vi "TEST Object Manual Bounds (Advanced By Reference Splitter).vi"() -> ()   [LabVIEW 2021, in "IObject.lvclass"]
uses:
  IObject.lvclass
  Object/Object.lvclass
  C:/Projects/Dynamic-Scaling/Dynamic Scaling/IObject.lvclass
  IContainer/Viewport/Viewport.lvclass
  IContainer/Divider/Splitter/Splitter.lvclass
  Interaction By Refererence/Interaction By Refererence.lvclass
panel:
  out "XY Graph 6":cluster{"X":dbl, "Y":dbl}[](graph)
  out "XY Graph 5":cluster{"X":dbl, "Y":dbl}[](graph)
  out "XY Graph 4":cluster{"X":dbl, "Y":dbl}[](graph)
  out "XY Graph 3":cluster{"X":dbl, "Y":dbl}[](graph)
  out "XY Graph 2":cluster{"X":dbl, "Y":dbl}[](graph)
  out "XY Graph":cluster{"X":dbl, "Y":dbl}[](graph)
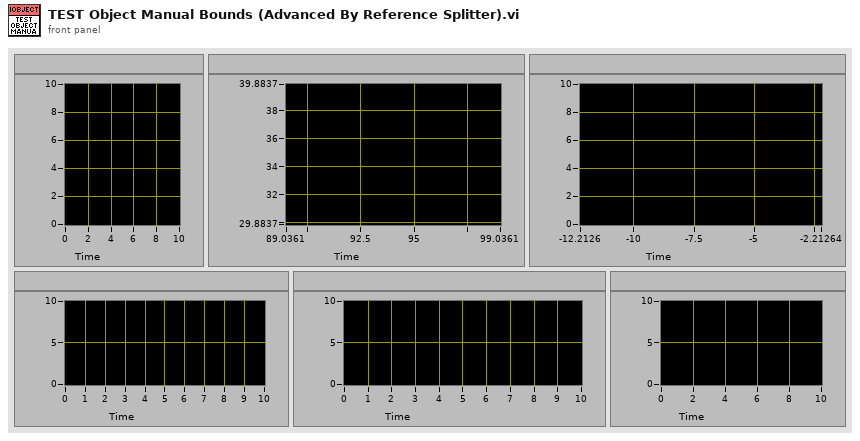
[diagram p1: front panel]
types:
  T1 = cluster{"Left":dbl, "Top":dbl, "Right":dbl, "Bottom":dbl}
  T2 = typedef "LVRectTypeDef.ctl" = cluster{"Left":i16, "Top":i16, "Right":i16, "Bottom":i16}
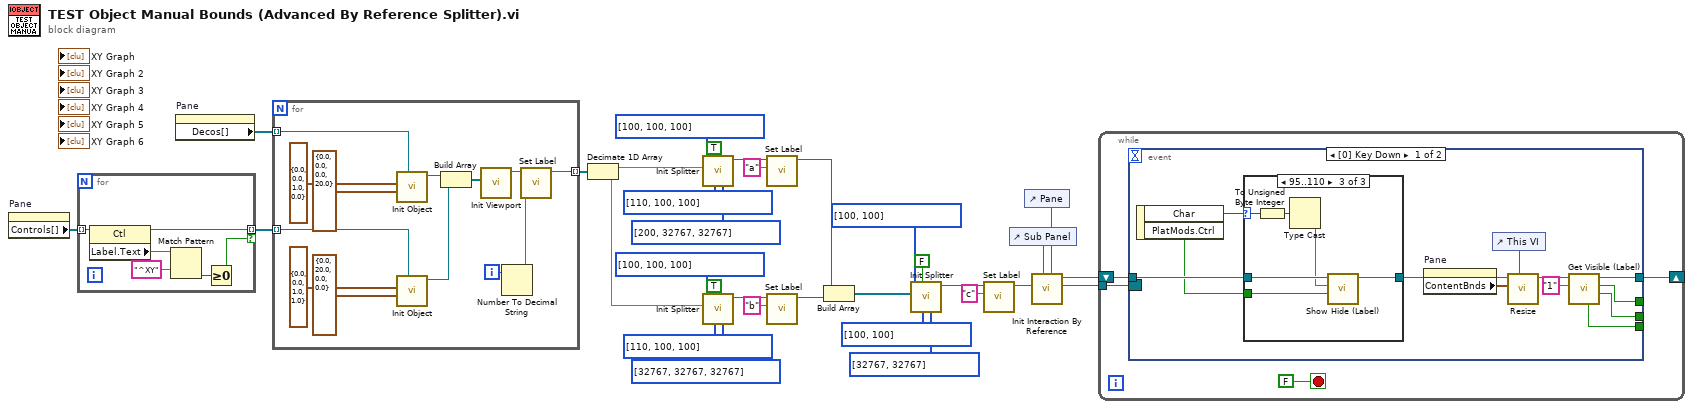
[diagram p0: block diagram]
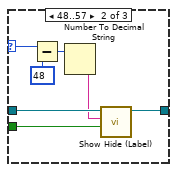
[diagram p3: hidden frame]
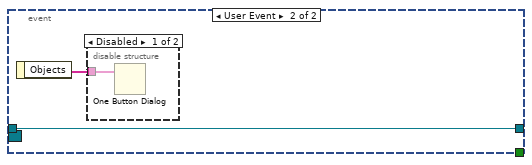
[diagram p4: hidden frame]
diagram:
  n1 = property on="Pane" class="Pane"() -> ("Controls[]"=w6:refnum<vi>[])  [unwired: 2 in, 2 out]
  n2 = for {
    tunnel: w6 -> [w38] mode=indexing
    tunnel: [w35] -> w5 mode=indexing if=w33
    n3 = property class="Ctl"(reference=w38) -> (reference out=w35:refnum<vi>, "Label.Text"=w37:string)  [unwired: 1 in, 1 out]
    n4 = Match Pattern(string=w37, regular expression="^XY") -> (offset past match=w34:i32)  [unwired: 1 in, 3 out]
    n5 = Greater Or Equal To 0?(x=w34) -> (x >= 0?=w33:bool)
  }
  n6 = property on="Pane" class="Pane"() -> ("Decos[]"=w30:refnum<vi>[])  [unwired: 2 in, 2 out]
  n7 = for {
    tunnel: w30 -> [w51] mode=indexing
    tunnel: [w40] -> w24 mode=indexing
    tunnel: w5 -> [w44] mode=indexing
    i -> [w50]
    n8 = call "Init Object.vi"("GObj Refnum"=w51, "B [0, 0, 0, 0]"=T1 {"Left"=0.0, "Top"=0.0, "Right"=0.0, "Bottom"=20.0} ("B"), "A [0, 0, 1, 1]"=T1 {"Left"=0.0, "Top"=0.0, "Right"=1.0, "Bottom"=0.0} ("A")) -> ("MMI Scaling out"=w42:refnum<class "Object.lvclass">)  [unwired: 7 in, 1 out]
    n9 = call "Init Object.vi"("GObj Refnum"=w44, "B [0, 0, 0, 0]"=T1 {"Left"=0.0, "Top"=20.0, "Right"=0.0, "Bottom"=0.0} ("B"), "A [0, 0, 1, 1]"=T1 {"Left"=0.0, "Top"=0.0, "Right"=1.0, "Bottom"=1.0} ("A")) -> ("MMI Scaling out"=w41:refnum<class "Object.lvclass">)  [unwired: 7 in, 1 out]
    n10 = Build Array(w42, w41) -> (w47:refnum<class "Object.lvclass">[])
    n11 = call "Init Viewport.vi"("Items"=w47) -> ("Viewport out"=w39:refnum<class "Viewport.lvclass">)  [unwired: 9 in, 1 out]
    n12 = Number To Decimal String(number=w50) -> (decimal integer string=w43:string)  [unwired: 1 in]
    n13 = call "Set Label.vi"("Label"=w43, "MMI Scaling in"=w39) -> ("MMI Scaling out"=w40:refnum<class "Viewport.lvclass">)  [unwired: 8 in, 1 out]
  }
  n14 = Decimate 1D Array(w24) -> (w25:refnum<class "Viewport.lvclass">[], w17:refnum<class "Viewport.lvclass">[])
  n15 = call "Init Splitter.vi"("Maximal size"=i16[] [200, 32767, 32767] ("Minimal size"), "Minimal size"=i16[] [110, 100, 100], "Vertical? [F, hor.]"=TRUE, "Relative size"=i16[] [100, 100, 100] ("Minimal size"), "Items"=w25) -> ("Splitter out"=w32:refnum<class "Splitter.lvclass">)  [unwired: 5 in, 1 out]
  n16 = call "Init Splitter.vi"("Maximal size"=i16[] [32767, 32767, 32767] ("Minimal size"), "Minimal size"=i16[] [110, 100, 100], "Vertical? [F, hor.]"=TRUE, "Relative size"=i16[] [100, 100, 100] ("Minimal size"), "Items"=w17) -> ("Splitter out"=w18:refnum<class "Splitter.lvclass">)  [unwired: 5 in, 1 out]
  n17 = call "Set Label.vi"("Label"="a", "MMI Scaling in"=w32) -> ("MMI Scaling out"=w14:refnum<class "Splitter.lvclass">)  [unwired: 8 in, 1 out]
  n18 = call "Set Label.vi"("Label"="b", "MMI Scaling in"=w18) -> ("MMI Scaling out"=w16:refnum<class "Splitter.lvclass">)  [unwired: 8 in, 1 out]
  n19 = Build Array(w14, w16) -> (w15:refnum<class "Splitter.lvclass">[])
  n20 = call "Init Splitter.vi"("Maximal size"=i16[] [32767, 32767] ("Size"), "Minimal size"=i16[] [100, 100] ("Size"), "Vertical? [F, hor.]"=FALSE, "Relative size"=i16[] [100, 100] ("Size"), "Items"=w15) -> ("Splitter out"=w8:refnum<class "Splitter.lvclass">)  [unwired: 5 in, 1 out]
  n21 = call "Set Label.vi"("Label"="c", "MMI Scaling in"=w8) -> ("MMI Scaling out"=w7:refnum<class "Splitter.lvclass">)  [unwired: 8 in, 1 out]
  n22 = control-ref of="Sub Panel"() -> (w4:refnum<vi>)
  n23 = control-ref of="Pane"() -> (w2:refnum<vi>)
  n24 = call "Init Interaction By Reference.vi"("Pane"=w2, "Sub Panel"=w4, "IObject"=w7) -> ("Object resize event"=w1:refnum<event-registration>, "Interaction out"=w3:refnum<class "Interaction By Refererence.lvclass">)  [unwired: 6 in, 1 out]
  n25 = while {
    shift-right: [w53] -> _
    shift-left: w3 -> [w55]
    tunnel: w1 -> [w52]
    stop <- FALSE stop-if-true
    n26 = event shown="[0] Key Down" {
      selector: w52 -> [_ _]
      dyn-events: _ -> [_ _]
      timeout: _ -> [_ _]
      tunnel: w55 -> [w63 w83]
      tunnel: [w60 w83] -> w53
      tunnel: [w58 _] -> _
      tunnel: [w57 _] -> _
      tunnel: [w56 _] -> _
      event Key Down {
        n27 = event-data() -> ("Char"=w65:i16, "PlatMods.Ctrl"=w62:bool)  [unwired: 1 in]
        n28 = case shown="95..110" w65 {
          selector: w65 -> [_ w75 w79]
          tunnel: [w68 w71 w80] -> w64
          tunnel: w63 -> [w68 w73 w81]
          tunnel: w62 -> [_ w70 w77]
          frame Default {
          }
          frame 48..57 {
            n29 = Subtract(x=w75, y=i16 48) -> (x-y=w72:i16)
            n30 = Number To Decimal String(number=w72) -> (decimal integer string=w69:string)  [unwired: 1 in]
            n31 = call-dynamic "Show Hide (Label).vi"("Show? [T]"=w70, "Label"=w69, "MMI Scaling in"=w73) -> ("MMI Scaling out"=w71:refnum<class "Interaction By Refererence.lvclass">)  [unwired: 6 in, 2 out]
          }
          frame 95..110 {
            n32 = To Unsigned Byte Integer(number=w79) -> (unsigned 8bit integer=w78:u8)
            n33 = Type Cast(x=w78) -> (*(type *) &x=w76:string)  [unwired: 1 in]
            n34 = call-dynamic "Show Hide (Label).vi"("Show? [T]"=w77, "Label"=w76, "MMI Scaling in"=w81) -> ("MMI Scaling out"=w80:refnum<class "Interaction By Refererence.lvclass">)  [unwired: 6 in, 2 out]
          }
        }
        n35 = property on="Pane" class="Pane"() -> ("ContentBnds"=w67:T2)  [unwired: 2 in, 2 out]
        n36 = control-ref of="This VI"() -> (w66:refnum<vi>)
        n37 = call-dynamic "Resize.vi"("VI Refnum"=w66, "Bounds"=w67, "MMI Scaling in"=w64) -> ("MMI Scaling out"=w61:refnum<class "Interaction By Refererence.lvclass">)  [unwired: 6 in, 2 out]
        n38 = call-dynamic "Get Visible (Label).vi"("Label"="1", "Interaction By Refererence in"=w61) -> ("Match?"=w57:bool, "Visible?"=w58:bool, "Interaction By Refererence out"=w60:refnum<class "Interaction By Refererence.lvclass">, "Item visible?"=w56:bool)  [unwired: 5 in, 1 out]
      }
      event User Event {
        n39 = event-data() -> ("Objects"=w82:string[])  [unwired: 1 in]
        n40 = disable-structure shown="Disabled" {
          disable-tunnel: w82 -> [w84 _]
          frame Disabled {
            n41 = One Button Dialog(message=w84) -> ()  [unwired: 1 in, 1 out]
          }
          frame Enabled {
          }
        }
      }
    }
  }
